vi "SendRaw.vi"() -> ()   [LabVIEW 2015]
uses:
  <vilib>/rvi/Emulation/niFpgaGetClockAttributes.vi
  <vilib>/rvi/Emulation/niFpgaSctlEmulationGetInTimedLoop.vi
  <vilib>/rvi/Emulation/niFpgaEmulationReportErrorSimple.vi
  <vilib>/rvi/eio/common/nirviEmuTemplateMethod_errors.vi
  <vilib>/rvi/interface/RandomDataEmulation/niFpgaRandomDataHandleErrors.vi
  <vilib>/rvi/Emulation/niFpgaCriticalErrorInLSC.vi
  <vilib>/eio/EIONode/EIONode.xnode
  <vilib>/rvi/Analysis/measure/butterworth/XNode/niFpgaButterworthFilter.xnode
  <vilib>/rvi/DataTransferAndStorage/Container/XNode/niFpgaContainer.xnode
  <vilib>/rvi/interface/RandomDataEmulation/nirviRandomDataFpgaReadWriteTemplate.vi
panel:
  in  "Channel":i16=80
  in  "Raw":bool
  out "Input Raw":sgl(slide)=5.0 scale=-6.0..6.0
  in  "Input period (ticks)":i16=80
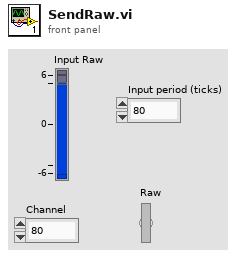
[diagram p1: front panel]
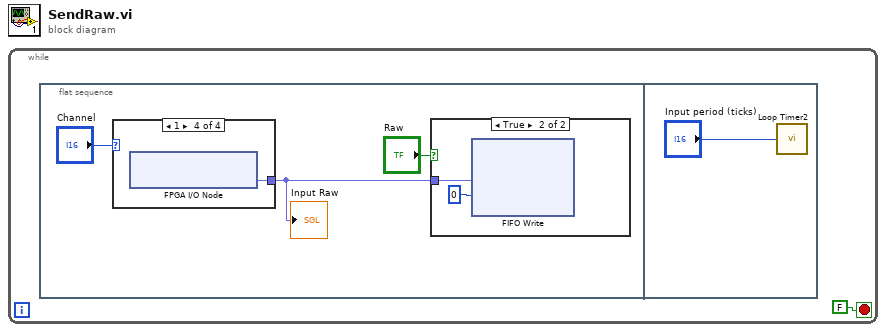
[diagram p0: block diagram]
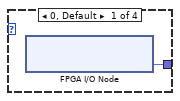
[diagram p2: hidden frame]
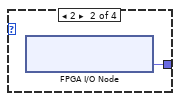
[diagram p3: hidden frame]
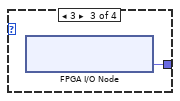
[diagram p4: hidden frame]
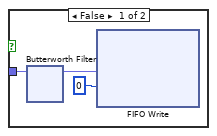
[diagram p5: hidden frame]
diagram:
  n1 = while {
    stop <- FALSE stop-if-true
    n2 = flat-sequence {
      frame #0 {
        n3 = case shown="1" "Channel" {
          tunnel: [w5 w6 w7 w8] -> w3
          frame 0, Default {
            n4 = xnode "FPGA I/O Node"() -> ("Connector0/AI0"=w5:fxp<+/-,27,5>)  [unwired: 1 in, 1 out]
          }
          frame 2 {
            n5 = xnode "FPGA I/O Node"() -> ("Connector0/AI2"=w6:fxp<+/-,27,5>)  [unwired: 1 in, 1 out]
          }
          frame 3 {
            n6 = xnode "FPGA I/O Node"() -> ("Connector0/AI3"=w7:fxp<+/-,27,5>)  [unwired: 1 in, 1 out]
          }
          frame 1 {
            n7 = xnode "FPGA I/O Node"() -> ("Connector0/AI1"=w8:fxp<+/-,27,5>)  [unwired: 1 in, 1 out]
          }
        }
        "Input Raw" <- w3
        n8 = case shown="True" "Raw" {
          tunnel: w3 -> [w10 w20]
          frame False {
            n9 = xnode "Butterworth Filter"("input data"=w10) -> ("output data"=w9:fxp<+/-,31,9>)  [unwired: 2 in]
            n10 = xnode ("FIFO Write")("Element"=w9, "Timeout"=i16 0) -> ()  [unwired: 1 in, 2 out]
          }
          frame True {
            n11 = xnode ("FIFO Write")("Element"=w20, "Timeout"=i16 0) -> ()  [unwired: 1 in, 2 out]
          }
        }
      }
      frame #1 {
        n12 = call "Loop Timer2"("Count(Ticks)"="Input period (ticks)") -> ()  [unwired: 1 out]
      }
    }
  }
